vi "719 SwitchBoard Demo.vi"() -> ()   [LabVIEW 2018]
uses:
  <vilib>/Modbus/master/Modbus Master.lvclass
  <vilib>/Modbus/master/Create Master Instance (TCP).vi
panel:
  out "Status":string
  in  "Device List":string(tree)
  in  "Switch Control":T1
  in  "QF Electric Parameter":string[][](table)
  in  "Connect":bool
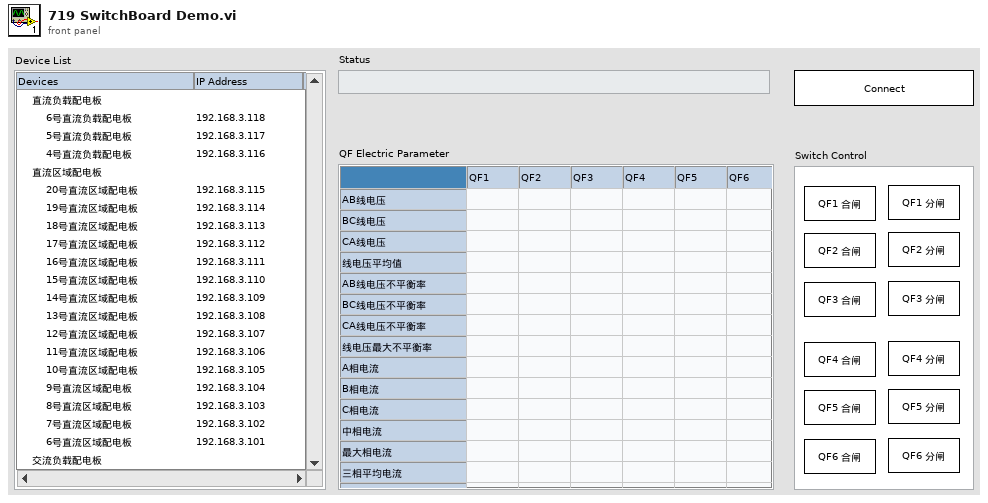
[diagram p1: front panel]
types:
  T1 = cluster{"合闸":bool, "分闸":bool, "合闸 2":bool, "分闸 2":bool, "合闸 3":bool, "分闸 3":bool, "合闸 4":bool, "分闸 4":bool, "合闸 5":bool, "分闸 5":bool, "合闸 6":bool, "分闸 6":bool}
  T2 = cluster{"TCP master instance":refnum<class "Modbus Master.lvclass">, "Device Name":string[], "IP Address":string[]}
  T3 = enum32{"invalid app kind", "Development System", "Run Time System", "Student Edition", "Embedded LabVIEW", "Evaluation", "Custom"}
  T4 = typedef "LVPoint32TypeDef.ctl" = cluster{"Horizontal":i32, "Vertical":i32}
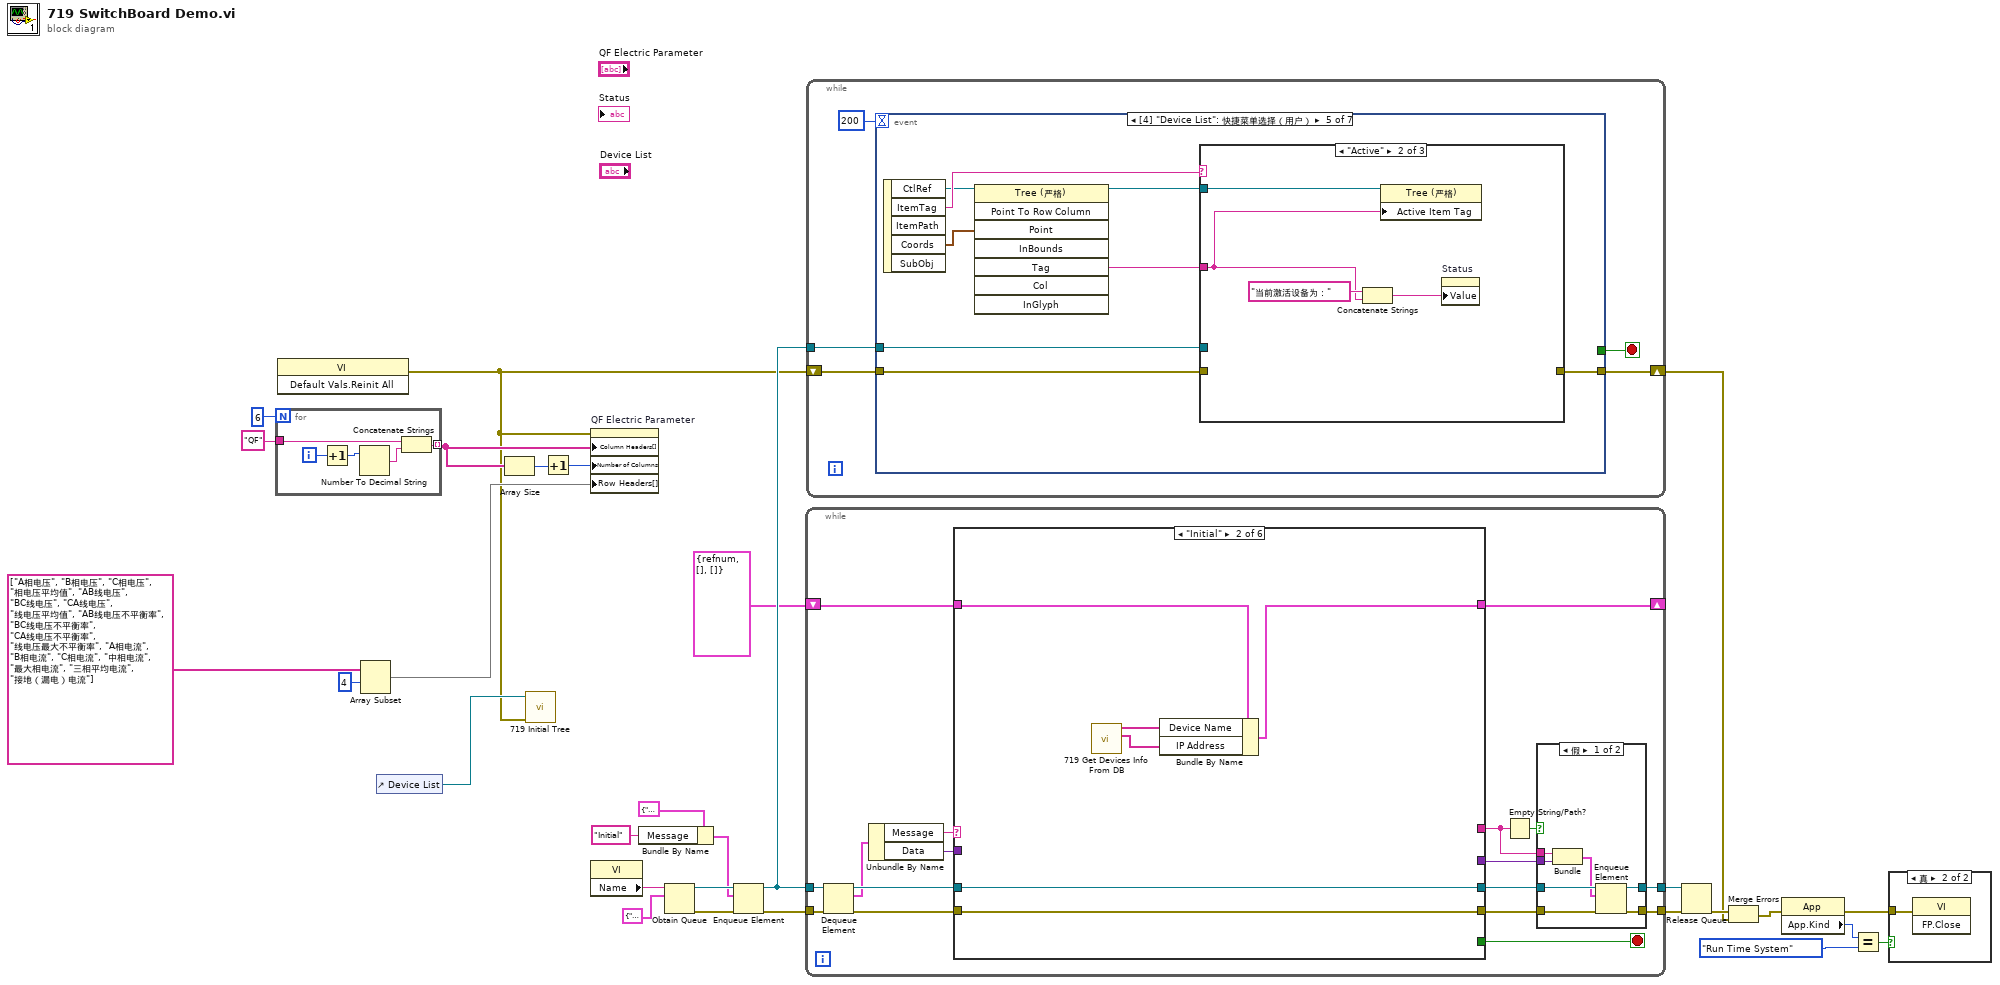
[diagram p0: block diagram]
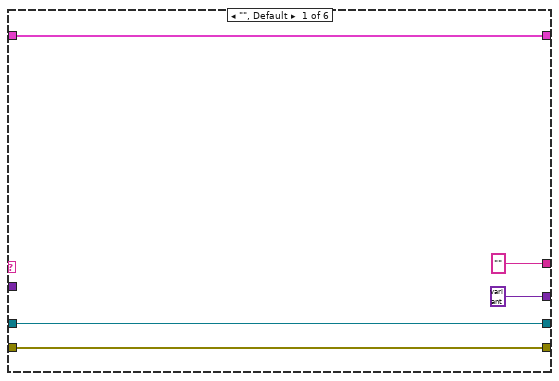
[diagram p4: hidden frame]
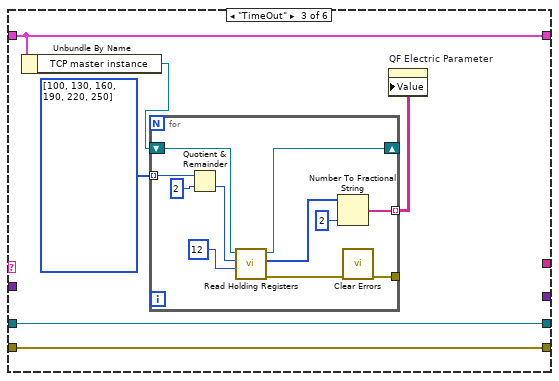
[diagram p5: hidden frame]
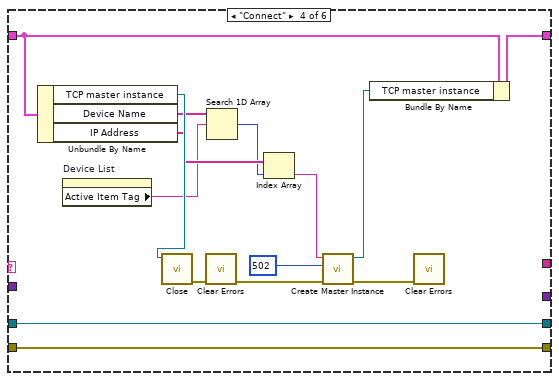
[diagram p6: hidden frame]
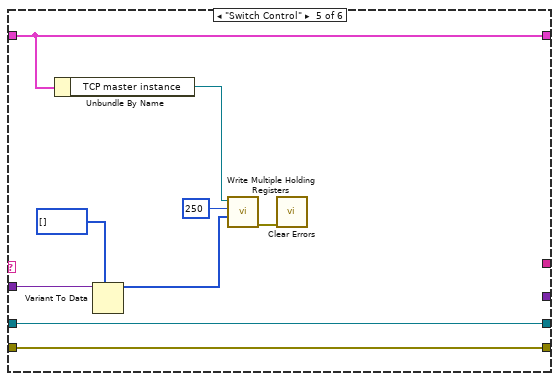
[diagram p7: hidden frame]
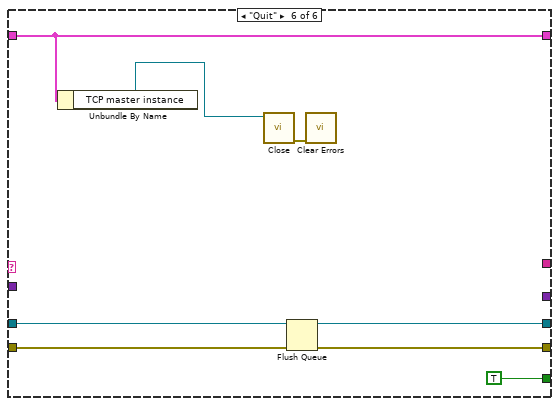
[diagram p8: hidden frame]
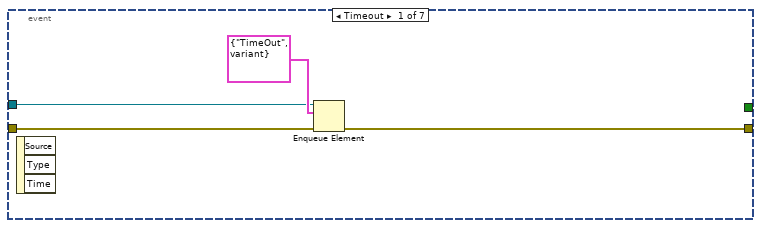
[diagram p9: hidden frame]
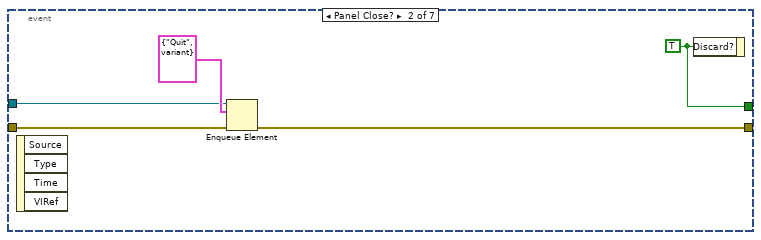
[diagram p10: hidden frame]
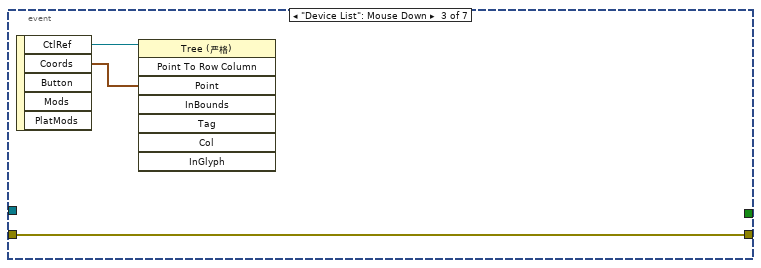
[diagram p11: hidden frame]
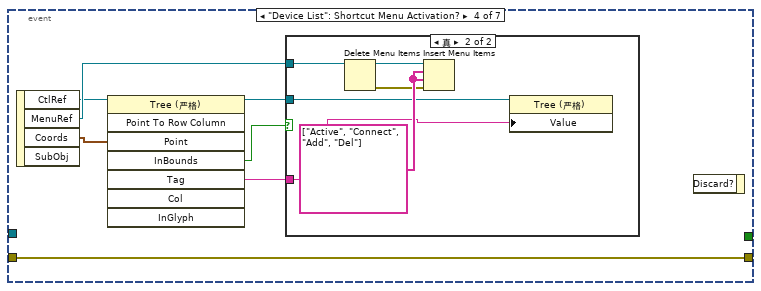
[diagram p12: hidden frame]
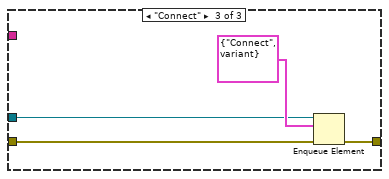
[diagram p15: hidden frame]
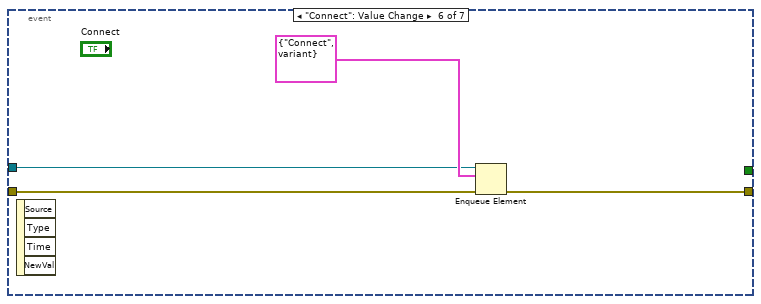
[diagram p16: hidden frame]
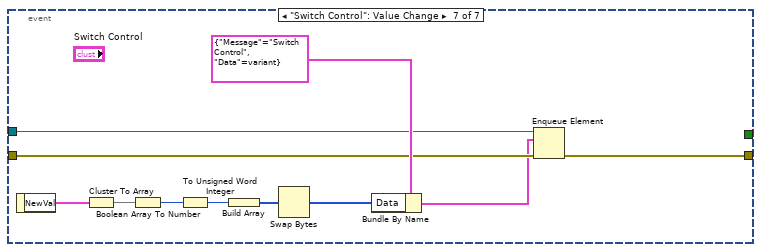
[diagram p17: hidden frame]
diagram:
  n1 = for {
    N: 6 -> [_]
    tunnel: "QF" -> [w32]
    tunnel: [w30] -> w23 mode=indexing
    i -> [w34]
    n2 = Increment(x=w34) -> (x+1=w33:i32)
    n3 = Number To Decimal String(number=w33) -> (decimal integer string=w31:string)  [unwired: 1 in]
    n4 = Concatenate Strings(w32, w31) -> (w30:string)
  }
  n5 = invoke class="VI" method="Default Vals.Reinit All"() -> (error out=w2:errorcluster)  [unwired: 3 in, 2 out]
  n6 = Array Subset(array=string[] ["A相电压", "B相电压", "C相电压", "相电压平均值", "AB线电压", "BC线电压", "CA线电压", "线电压平均值", "AB线电压不平衡率", "BC线电压不平衡率", "CA线电压不平衡率", "线电压最大不平衡率", "A相电流", "B相电流", "C相电流", "中相电流", "最大相电流", "三相平均电流", "接地（漏电）电流"] ("数组"), index=4 ("索引")) -> (w25:string[])  [unwired: 1 in]
  n7 = control-ref of="Device List"() -> (w3:refnum<vi>)
  n8 = Array Size(array=w23) -> (size(s)=w24:i32)
  n9 = call "719 Initial Tree.vi"("error in (no error)"=w2, "树形控件"=w3) -> ()  [unwired: 9 in, 1 out]
  n10 = Increment(x=w24) -> (x+1=w22:i32)
  n11 = property on="QF Electric Parameter" class="Tbl (严格)"(error in=w2, "Column Headers[]"=w23, "Number of Columns"=w22, "Row Headers[]"=w25) -> ()  [unwired: 1 in, 2 out]
  n12 = property class="VI"() -> ("Name"=w17:string)  [unwired: 2 in, 2 out]
  n13 = Bundle By Name(cluster=cluster{"Message":string, "Data":variant} {"Message"="", "Data"=variant}, "Message"="Initial") -> (w14:cluster{"Message":string, "Data":variant})
  n14 = Obtain Queue(name (unnamed)=w17, element data type=cluster{"Message":string, "Data":variant} {"Message"="", "Data"=variant}) -> (queue out=w19:refnum<queue>, error out=w18:errorcluster)  [unwired: 3 in, 1 out]
  n15 = Enqueue Element(queue=w19, element=w14, error in (no error)=w18) -> (queue out=w11:refnum<queue>, error out=w12:errorcluster)  [unwired: 1 in, 1 out]
  n16 = while {
    tunnel: w11 -> [w51]
    tunnel: [w40] -> w21
    tunnel: w12 -> [w49]
    tunnel: [w39] -> w20
    shift-right: [w35] -> _
    shift-left: T2 {"TCP master instance"=refnum, "Device Name"=[], "IP Address"=[]} ("输出簇") -> [w36]
    stop <- w47 stop-if-true
    n17 = Dequeue Element(queue=w51, error in (no error)=w49) -> (queue out=w50:refnum<queue>, element=w46:cluster{"Message":string, "Data":variant}, error out=w48:errorcluster)  [unwired: 1 in, 1 out]
    n18 = Unbundle By Name(w46) -> ("Message"=w45:string, "Data"=w44:variant)
    n19 = case shown="\"Initial\"" w45 {
      tunnel: w50 -> [w65 w71 w77 w103 w112 w120]
      tunnel: [w65 w71 w77 w103 w112 w118] -> w41
      tunnel: w48 -> [w64 w70 w76 w102 w111 w119]
      tunnel: [w64 w70 w76 w102 w111 w117] -> w42
      tunnel: [_ _ _ _ _ TRUE] -> w47
      tunnel: w44 -> [_ _ _ _ w105 _]
      tunnel: ["" _ _ _ _ _] -> w37
      tunnel: [variant _ _ _ _ _] -> w38
      tunnel: w36 -> [w61 w67 w74 w101 w108 w114]
      tunnel: [w61 w66 w74 w96 w108 w114] -> w35
      frame "", Default {
      }
      frame "Initial" {
        n20 = call "719 Get Devices Info From DB.vi"() -> ("IP Address"=w68:string[], "Device Name"=w69:string[])  [unwired: 8 in, 2 out]
        n21 = Bundle By Name(cluster=w67, "Device Name"=w69, "IP Address"=w68) -> (w66:T2)
      }
      frame "TimeOut" {
        n22 = Unbundle By Name(w74) -> ("TCP master instance"=w73:refnum<class "Modbus Master.lvclass">)
        n23 = for {
          shift-right: [w87] -> _
          shift-left: w73 -> [w88]
          tunnel: u16[] [100, 130, 160, 190, 220, 250] -> [w85] mode=indexing
          tunnel: [w81] -> _
          tunnel: [w79] -> w72 mode=indexing
          n24 = Quotient & Remainder(x=w85, y=u16 2) -> (floor(x/y)=w83:u16)  [unwired: 1 out]
          n25 = call-dynamic "Read Holding Registers.vi"("number of holding registers"=u16 12, "starting address"=w83, "Modbus master in"=w88) -> ("error out"=w82:errorcluster, "register values"=w80:u16[], "Modbus master out"=w87:refnum<class "Modbus Master.lvclass">)  [unwired: 6 in]
          n26 = Number To Fractional String(number=w80, precision (6)=i16 2 ("精度(6)")) -> (F-format string=w79:string[])  [unwired: 2 in]
          n27 = call <vilib>:"Clear Errors.vi"("error in (no error)"=w82) -> ("error out"=w81:errorcluster)  [unwired: 5 in, 1 out]
        }
        n28 = property on="QF Electric Parameter" class="Tbl (严格)"("Value"=w72) -> ()  [unwired: 2 in, 2 out]
      }
      frame "Connect" {
        n29 = Unbundle By Name(w101) -> ("TCP master instance"=w99:refnum<class "Modbus Master.lvclass">, "Device Name"=w91:string[], "IP Address"=w93:string[])
        n30 = property on="Device List" class="Tree (严格)"() -> ("Active Item Tag"=w90:string)  [unwired: 2 in, 2 out]
        n31 = call-dynamic "Close.vi"("Modbus master in"=w99) -> ("error out"=w100:errorcluster)  [unwired: 10 in]
        n32 = call <vilib>:"Clear Errors.vi"("error in (no error)"=w100) -> ("error out"=w97:errorcluster)  [unwired: 5 in, 1 out]
        n33 = Search 1D Array(1D array=w91, element=w90) -> (index of element=w89:i32)  [unwired: 1 in]
        n34 = Index Array(array=w93, index=w89) -> (element=w92:string)
        n35 = call-poly <vilib>:"Create Master Instance.vi"("error in (no error)"=w97, "port (502)"=u16 502, "address"=w92) -> ("error out"=w94:errorcluster, "TCP master instance"=w95:refnum<class "Modbus Master.lvclass">)  [unwired: 7 in]
        n36 = Bundle By Name(cluster=w101, "TCP master instance"=w95) -> (w96:T2)
        n37 = call <vilib>:"Clear Errors.vi"("error in (no error)"=w94) -> ()  [unwired: 5 in, 2 out]
      }
      frame "Switch Control" {
        n38 = Unbundle By Name(w108) -> ("TCP master instance"=w107:refnum<class "Modbus Master.lvclass">)
        n39 = Variant To Data(type=u16[] [] ("holding register values"), Variant=w105) -> (data=w104:u16[])  [unwired: 1 in, 1 out]
        n40 = call-dynamic "Write Multiple Holding Registers.vi"("holding register values"=w104, "starting address"=u16 250, "Modbus master in"=w107) -> ("error out"=w109:errorcluster)  [unwired: 7 in, 1 out]
        n41 = call <vilib>:"Clear Errors.vi"("error in (no error)"=w109) -> ()  [unwired: 5 in, 2 out]
      }
      frame "Quit" {
        n42 = Unbundle By Name(w114) -> ("TCP master instance"=w113:refnum<class "Modbus Master.lvclass">)
        n43 = call-dynamic "Close.vi"("Modbus master in"=w113) -> ("error out"=w115:errorcluster)  [unwired: 10 in]
        n44 = Flush Queue(queue=w120, error in (no error)=w119) -> (queue out=w118:refnum<queue>, error out=w117:errorcluster)  [unwired: 1 out]
        n45 = call <vilib>:"Clear Errors.vi"("error in (no error)"=w115) -> ()  [unwired: 5 in, 2 out]
      }
    }
    n46 = Empty String/Path?(string/path=w37) -> (empty?=w43:bool)
    n47 = case shown="假" w43 {
      tunnel: w42 -> [w58 w59]
      tunnel: w41 -> [w57 w60]
      tunnel: [w55 w60] -> w40
      tunnel: [w54 w59] -> w39
      tunnel: w37 -> [w53 _]
      tunnel: w38 -> [w52 _]
      frame False {
        n48 = Bundle(w53, w52) -> (w56:cluster{string, variant})  [unwired: 1 in]
        n49 = Enqueue Element(queue=w57, element=w56, error in (no error)=w58) -> (queue out=w55:refnum<queue>, error out=w54:errorcluster)  [unwired: 1 in, 1 out]
      }
      frame True {
      }
    }
  }
  n50 = while {
    shift-right: [w124] -> w4
    shift-left: w2 -> [w125]
    tunnel: w11 -> [w121]
    stop <- w122 stop-if-true
    n51 = event shown="[4] \"Device List\": 快捷菜单选择（用户）" {
      selector: _ -> [_ _ _ _ _ _ _]
      dyn-events: _ -> [_ _ _ _ _ _ _]
      timeout: 200 -> [_ _ _ _ _ _ _]
      tunnel: w125 -> [w127 w131 w137 w144 w156 w169 w176]
      tunnel: [w126 w130 w137 w144 w155 w168 w175] -> w124
      tunnel: [_ w134 _ _ _ _ _] -> w122
      tunnel: w121 -> [w128 w132 _ _ w157 w170 w174]
      event Timeout {
        n52 = event-data() -> ()  [unwired: 1 in, 3 out]
        n53 = Enqueue Element(queue=w128, element=cluster{"Message":string, "Data":variant} {"Message"="TimeOut", "Data"=variant}, error in (no error)=w127) -> (error out=w126:errorcluster)  [unwired: 1 in, 2 out]
      }
      event Panel Close? {
        w134 = TRUE ("放弃？")
        n54 = event-data() -> ()  [unwired: 1 in, 4 out]
        n55 = Enqueue Element(queue=w132, element=cluster{"Message":string, "Data":variant} {"Message"="Quit", "Data"=variant}, error in (no error)=w131) -> (error out=w130:errorcluster)  [unwired: 1 in, 2 out]
        n56 = event-data("Discard?"=w134) -> ()  [unwired: 1 in, 1 out]
      }
      event "Device List": Mouse Down {
        n57 = event-data() -> ("CtlRef"=w136:refnum<vi>, "Coords"=w135:T4)  [unwired: 1 in, 3 out]
        n58 = invoke class="Tree (严格)" method="Point To Row Column"(reference=w136, "Point"=w135) -> ()  [unwired: 6 in, 8 out]
      }
      event "Device List": Shortcut Menu Activation? {
        n59 = event-data() -> ("CtlRef"=w142:refnum<vi>, "MenuRef"=w143:refnum<k9>, "Coords"=w141:T4)  [unwired: 1 in, 1 out]
        n60 = invoke class="Tree (严格)" method="Point To Row Column"(reference=w142, "Point"=w141) -> (reference out=w138:refnum<vi>, "InBounds"=w140:bool, "Tag"=w139:string)  [unwired: 6 in, 5 out]
        n61 = case shown="真" w140 {
          tunnel: w143 -> [_ w150]
          tunnel: w139 -> [_ w146]
          tunnel: w138 -> [_ w147]
          frame False {
          }
          frame True {
            w148 = string[] ["Active", "Connect", "Add", "Del"] ("项名称")
            n62 = Delete Menu Items(9:w150) -> (0:w145:errorcluster, 3:w149:refnum<k9>)  [unwired: 3 in]
            n63 = Insert Menu Items(6:w145, 7:w148, 8:w148, 9:w149) -> ()  [unwired: 2 in, 3 out]
            n64 = property class="Tree (严格)"(reference=w147, "Value"=w146) -> ()  [unwired: 1 in, 2 out]
          }
        }
        n65 = event-data() -> ()  [unwired: 2 in, 1 out]
      }
      event "Device List": Shortcut Menu Selection (User) {
        n66 = event-data() -> ("CtlRef"=w154:refnum<vi>, "ItemTag"=w158:string, "Coords"=w153:T4)  [unwired: 1 in, 2 out]
        n67 = invoke class="Tree (严格)" method="Point To Row Column"(reference=w154, "Point"=w153) -> (reference out=w151:refnum<vi>, "Tag"=w152:string)  [unwired: 6 in, 6 out]
        n68 = case shown="\"Active\"" w158 {
          tunnel: w157 -> [_ _ w166]
          tunnel: w156 -> [w159 _ w165]
          tunnel: [w159 _ w164] -> w155
          tunnel: w152 -> [_ w161 _]
          tunnel: w151 -> [_ w163 _]
          frame "假", Default {
          }
          frame "Active" {
            n69 = Concatenate Strings("当前激活设备为：" ("字符串"), w161) -> (w160:string)
            n70 = property on="属性节点" class="Tree (严格)"(reference=w163, "Active Item Tag"=w161) -> ()  [unwired: 1 in, 2 out]
            n71 = property on="Status" class="Str"("Value"=w160) -> ()  [unwired: 2 in, 2 out]
          }
          frame "Connect" {
            n72 = Enqueue Element(queue=w166, element=cluster{"Message":string, "Data":variant} {"Message"="Connect", "Data"=variant}, error in (no error)=w165) -> (error out=w164:errorcluster)  [unwired: 1 in, 2 out]
          }
        }
      }
      event "Connect": Value Change {
        n73 = event-data() -> ()  [unwired: 1 in, 4 out]
        n74 = Enqueue Element(queue=w170, element=cluster{"Message":string, "Data":variant} {"Message"="Connect", "Data"=variant}, error in (no error)=w169) -> (error out=w168:errorcluster)  [unwired: 1 in, 2 out]
      }
      event "Switch Control": Value Change {
        n75 = event-data() -> ("NewVal"=w178:T1)  [unwired: 1 in]
        n76 = Cluster To Array(cluster=w178) -> (array=w182:bool[])
        n77 = Boolean Array To Number(Boolean array=w182) -> (number=w181:u32)
        n78 = To Unsigned Word Integer(number=w181) -> (unsigned 16bit integer=w179:u16)
        n79 = Build Array(w179) -> (w180:u16[])
        n80 = Swap Bytes(anything=w180) -> (byte swapped=w172:u16[])
        n81 = Bundle By Name(cluster=cluster{"Message":string, "Data":variant} {"Message"="Switch Control", "Data"=variant}, "Data"=w172) -> (w173:cluster{"Message":string, "Data":variant})
        n82 = Enqueue Element(queue=w174, element=w173, error in (no error)=w176) -> (error out=w175:errorcluster)  [unwired: 1 in, 2 out]
      }
    }
  }
  n83 = Release Queue(queue=w21, error in (no error)=w20) -> (error out=w6:errorcluster)  [unwired: 1 in, 2 out]
  n84 = Merge Errors(w6, w4) -> (w5:errorcluster)
  n85 = property class="App"(error in=w5) -> (error out=w7:errorcluster, "App.Kind"=w10:T3)  [unwired: 1 in, 1 out]
  n86 = Equal?(x=w10, y=T3."Run Time System" ("应用程序:类别")) -> (x = y?=w8:bool)
  n87 = case shown="真" w8 {
    tunnel: w7 -> [_ w183]
    frame False {
    }
    frame True {
      n88 = invoke class="VI" method="FP.Close"(error in=w183) -> ()  [unwired: 2 in, 3 out]
    }
  }
